vi "Channel or group name to index.vi"(0 "Name":string) -> (4 "Index":i32, 6 "Crate":i32, 8 "Card.Channel":dbl, 10 "Group":bool, 15 "error out":errorcluster)   [LabVIEW 2018]
uses:
  CAEN globals.vi
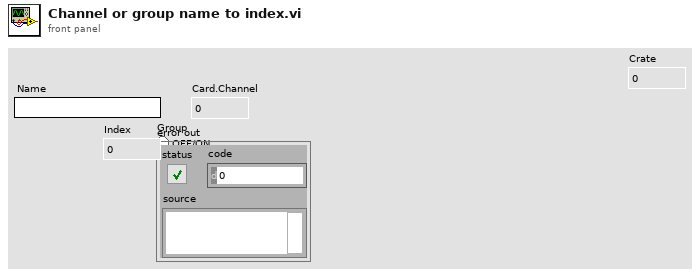
[diagram p1: front panel]
types:
  T1 = typedef "channel.ctl" = cluster{" Card.Channel":dbl, "Crate":i32}
  T2 = cluster{"Group Name":string, "Channels in Group":T1[]}[]
  T3 = typedef "channel_cluster.ctl" = cluster{"Channel Name":string, "Crate":i32, "Card Type":string, "Card":i32, "Channel":i32, "Status Icon":picture, "Vmon (V)":dbl, "Vset (V)":dbl, "Imon (A)":dbl, "Iset (A)":dbl, "Timestamp":string, "ON/OFF":bool, "Status":string, "Vswmax (V)":dbl, "Flag":bool, "Vfile (V)":dbl, "Error Logged":bool[], "enable_file":bool}
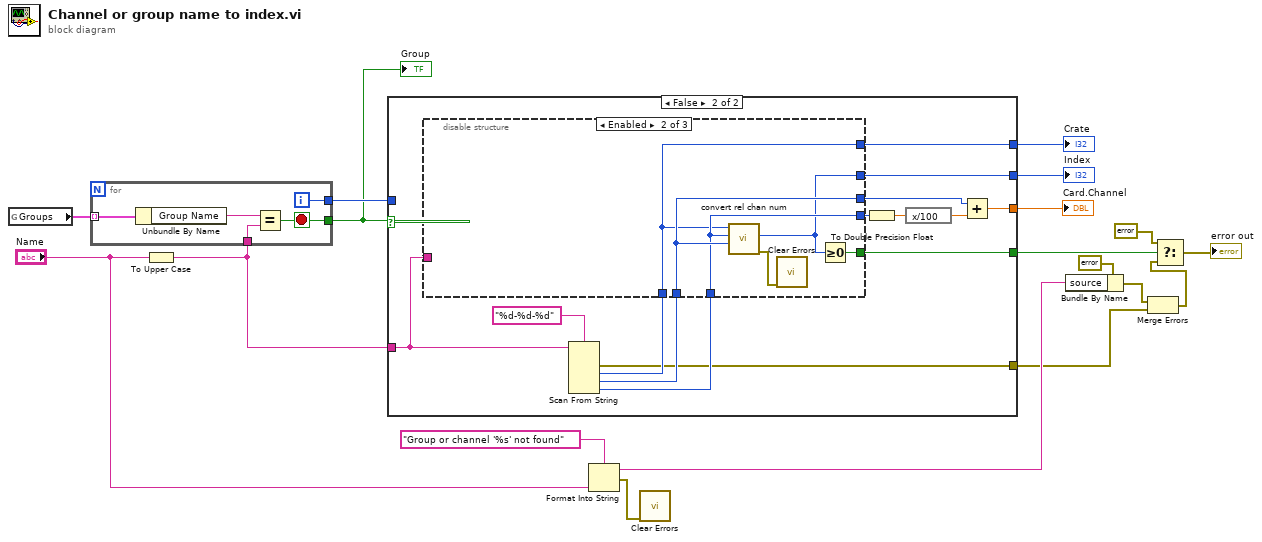
[diagram p0: block diagram]
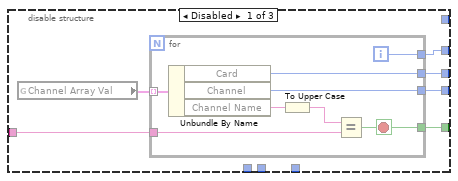
[diagram p3: hidden frame]
diagram:
  n1 = global read "CAEN globals.vi" "Groups"() -> (w18:T2)
  n2 = To Upper Case(1:"Name") -> (0:w10:string)
  n3 = for {
    tunnel: w18 -> [w23] mode=indexing
    tunnel: w10 -> [w21]
    tunnel: [w20] -> w17
    tunnel: [w19] -> w16
    i -> [w20]
    stop <- w19 stop-if-true
    n4 = Unbundle By Name(w23) -> ("Group Name"=w22:string)
    n5 = Equal?(x=w22, y=w21) -> (x = y?=w19:bool)
  }
  "Group" <- w16
  n6 = case shown="False" w16 {
    selector: w16 -> [w25 _]
    tunnel: w10 -> [_ w32]
    tunnel: [_ w35] -> w12
    tunnel: w17 -> [w24 _]
    tunnel: [w25 w34] -> w15
    tunnel: [w24 w33] -> w11
    tunnel: [_ w27] -> w9
    tunnel: [_ w26] -> w2
    frame True {
    }
    frame False {
      n7 = Scan From String(format string="%d-%d-%d", input string=w32) -> (error out=w26:errorcluster, output 1=w28:i32, output 2=w29:i32, output 3=w30:i32)  [unwired: 5 in, 2 out]
      n8 = disable-structure shown="Enabled" {
        disable-tunnel: [w45 w56 w61] -> w38
        disable-tunnel: [w44 w57 w60] -> w36
        disable-tunnel: [w43 w58 _] -> w34
        disable-tunnel: [w42 w54 _] -> w33
        disable-tunnel: w32 -> [w41 _ _]
        disable-tunnel: w30 -> [_ w56 w61]
        disable-tunnel: w29 -> [_ w57 w60]
        disable-tunnel: w28 -> [_ w55 _]
        disable-tunnel: [_ w55 _] -> w27
        frame Disabled {
          n9 = global read "CAEN globals.vi" "Channel Array Val"() -> (w40:T3[])
          n10 = for {
            tunnel: w40 -> [w53] mode=indexing
            tunnel: w41 -> [w52]
            tunnel: [w51] -> w45
            tunnel: [w50] -> w44
            tunnel: [w49] -> w43
            tunnel: [w48] -> w42
            i -> [w48]
            stop <- w49 stop-if-true
            n11 = Unbundle By Name(w53) -> ("Card"=w50:i32, "Channel"=w51:i32, "Channel Name"=w47:string)
            n12 = To Upper Case(1:w47) -> (0:w46:string)
            n13 = Equal?(x=w46, y=w52) -> (x = y?=w49:bool)
          }
        }
        frame Enabled {
          n14 = call "convert rel chan num.vi"("Card"=w57, "Channel"=w56, "Crate"=w55) -> ("error out"=w59:errorcluster, "Absolute index"=w54:i32)  [unwired: 5 in, 2 out]
          n15 = call <vilib>:"Clear Errors.vi"("error in (no error)"=w59) -> ()  [unwired: 5 in, 2 out]
          n16 = Greater Or Equal To 0?(x=w54) -> (x >= 0?=w58:bool)
        }
        frame Disabled {
        }
      }
      n17 = To Double Precision Float(number=w38) -> (double precision float=w39:dbl)
      n18 = expression code="x/100"(w39) -> (w37:dbl)
      n19 = Add(x=w36, y=w37) -> (x+y=w35:dbl)
    }
  }
  "Card.Channel" <- w12
  "Index" <- w11
  "Crate" <- w9
  n20 = Format Into String(format string="Group or channel '%s' not found" ("source"), "Name") -> (resulting string=w7:string, error out=w6:errorcluster)  [unwired: 2 in]
  n21 = call <vilib>:"Clear Errors.vi"("error in (no error)"=w6) -> ()  [unwired: 5 in, 2 out]
  n22 = Bundle By Name(cluster=errorcluster {"status"=TRUE, "code"=0, "source"=""} ("error out"), "source"=w7) -> (w3:errorcluster)
  n23 = Merge Errors(w3, w2) -> (w1:errorcluster)
  n24 = Select(t=errorcluster {"status"=FALSE, "code"=0, "source"=""}, s=w15, f=w1) -> (s? t:f=→"error out":errorcluster)
